vi "Glimpse Plugin Handler.vi"() -> ()   [LabVIEW 2016]
doc: "Select a listed SubVI (stand-alone or inside an .llb) and execute it. Plug-ins run asynchronously from Glimpse (this means that both the plug-in and Glimpse run simultaneously). Be careful about doing 2 things at once if one of the tasks is time-criticial (i.e., image acquisition).\n\nFor a plug-in to be included in the list, it must have the right name and be in the right place:\n-- the name must start with \"GPI-\" and end with \".vi\"\n-- for the executable version of Glimpse, plug-ins must be built into the installer; you can't add them later. (Specifically, the plug-in must be linked into the glimpse build as a dynamic VI to be placed in the installation directory.) The executable version of Glimpse also requres that each plug in be added to the list on the front panel of glimpse plugin list plugins.vi\n-- for the source version, the plug-in is simply placed in the same directory as Glimpse.llb\n\nGlimpse Plugin Handler.vi - created 8-3-05 by Marc Bunin\nmods JG 1/3/06"
panel:
  in  "error in (no error)":errorcluster
  out "stripped path":path
  in  "Execute":bool caption="Runs the selected SubVI and ends execution of the Plugin Handler."
  in  "Available Plug-ins":i32(listbox) caption="Select a VI and press Execute."
  in  "Cancel":bool caption="Stops execution of the Plugin Handler."
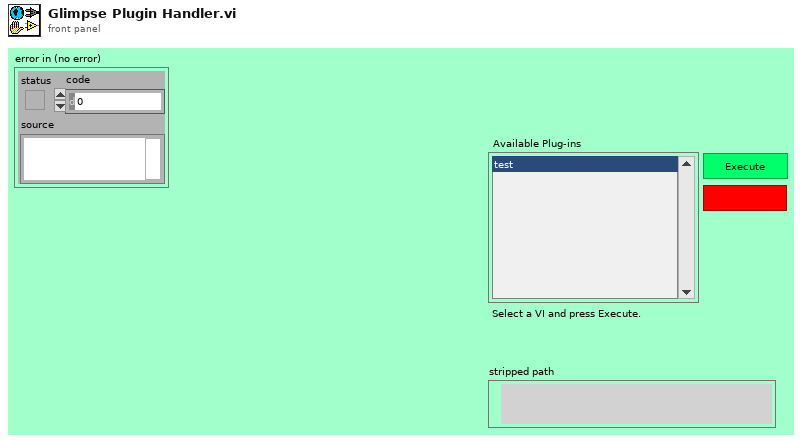
[diagram p1: front panel]
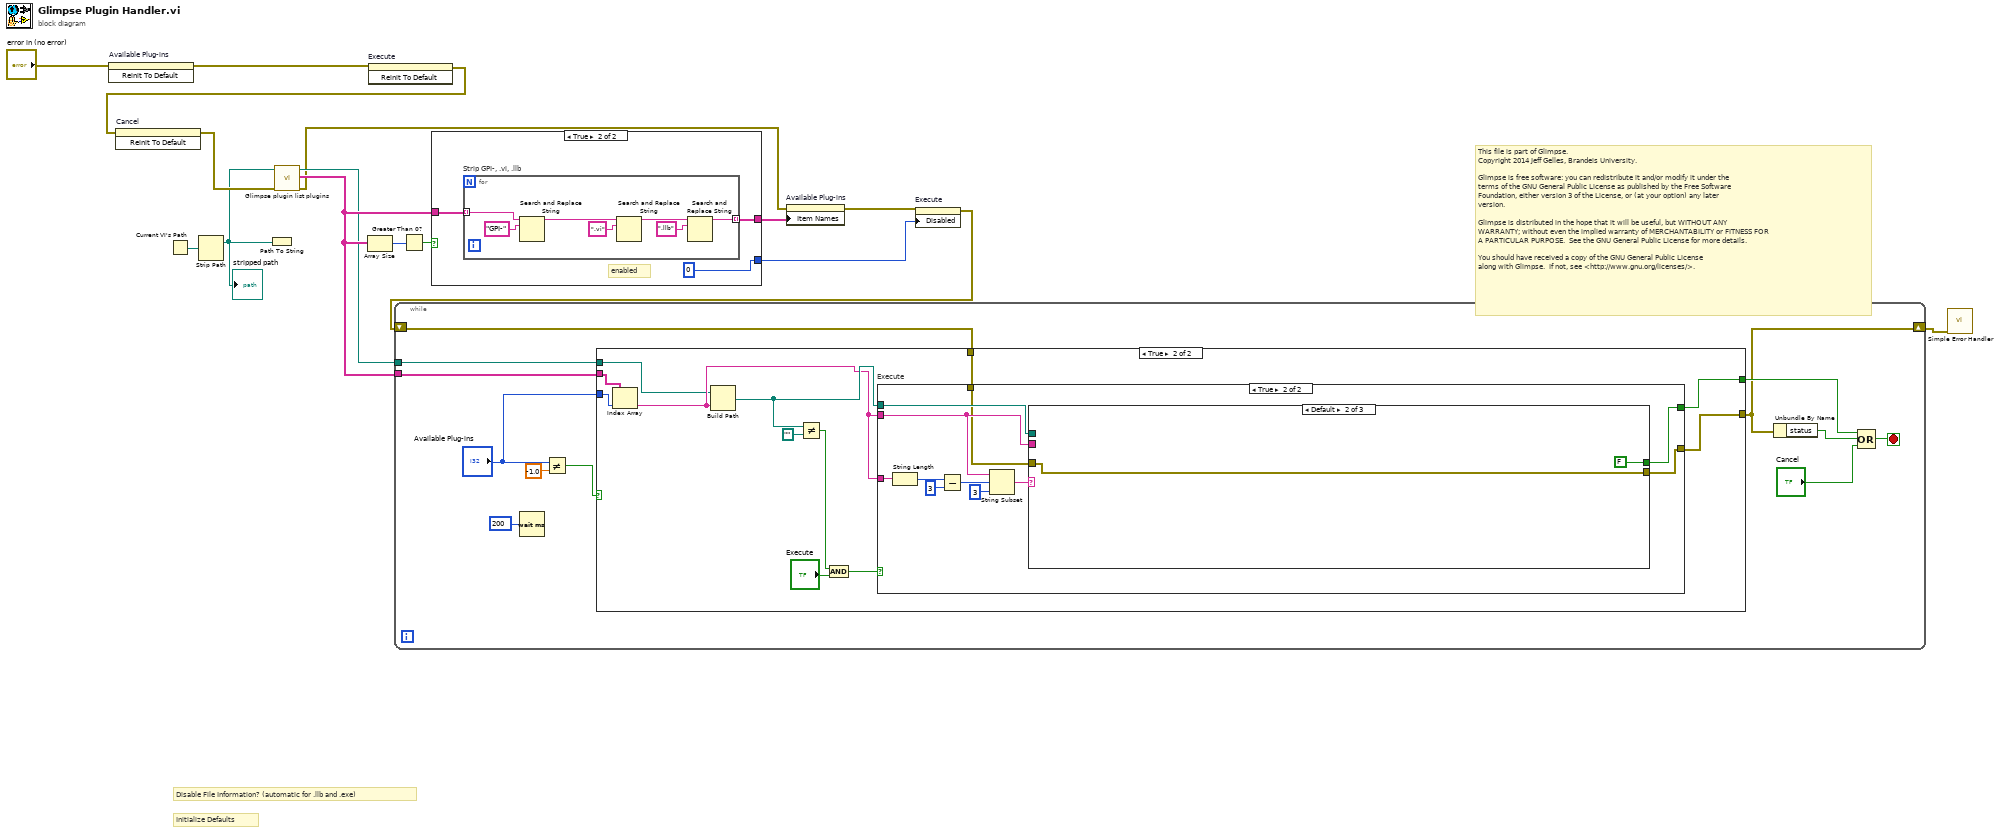
[diagram p0: block diagram]
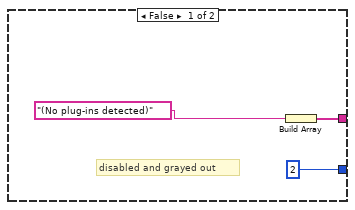
[diagram p2: hidden frame]
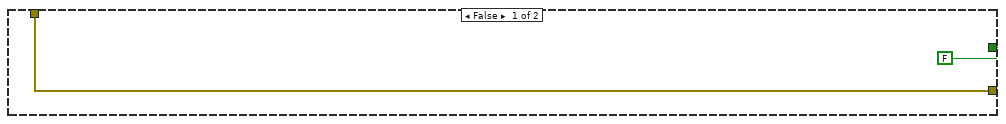
[diagram p3: hidden frame]
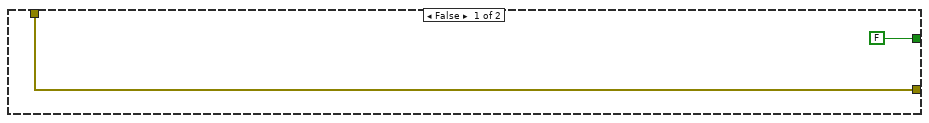
[diagram p4: hidden frame]
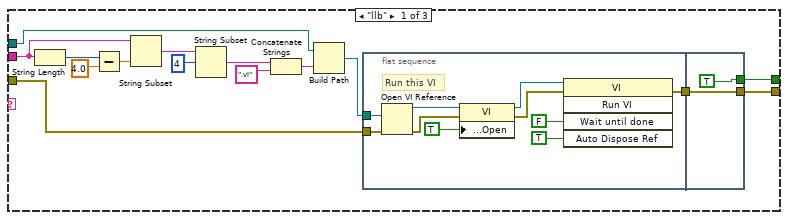
[diagram p5: hidden frame]
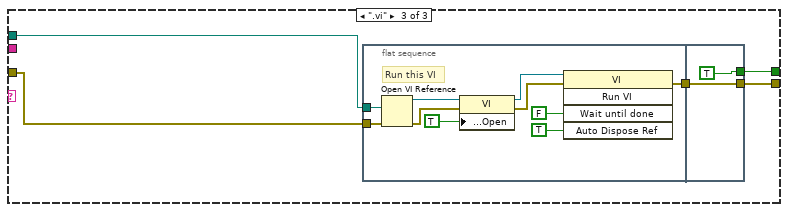
[diagram p6: hidden frame]
diagram:
  # "This file is part of Glimpse. \nCopyright 2014 Jeff Gelles, Brandeis University.    \n\nGlimpse is free software: you can redistribute it and/or modify it under the \nterms of the GNU General Public License as published by the Free Software \nFoundation, either version 3 of the License, or (at your option) any later \nversion.\n\nGlimpse is distributed in the hope that it will be useful, but WITHOUT ANY \nWARRANTY; without even the implied warranty of MERCHANTABILITY or FITNESS FOR \nA PARTICULAR PURPOSE.  See the GNU General Public License for more details.\n\nYou should have received a copy of the GNU General Public License\nalong with Glimpse.  If not, see <http://www.gnu.org/licenses/>."
  # "Disable File Information? (automatic for .llb and .exe)"
  # "Initialize Defaults"
  n1 = invoke on="Available Plug-ins" class="ListBox (strict)" method="Reinit To Default"(error in="error in (no error)") -> (error out=w5:errorcluster)  [unwired: 2 in, 2 out]
  n2 = Current VI's Path() -> (path=w16:path)
  n3 = Strip Path(path=w16) -> (stripped path=w7:path)  [unwired: 1 out]
  "stripped path" <- w7
  n4 = Path To String(path=w7) -> ()  [unwired: 1 out]
  n5 = invoke on="Execute" class="Boolean" method="Reinit To Default"(error in=w5) -> (error out=w15:errorcluster)  [unwired: 2 in, 2 out]
  n6 = invoke on="Cancel" class="Boolean" method="Reinit To Default"(error in=w15) -> (error out=w14:errorcluster)  [unwired: 2 in, 2 out]
  n7 = call "Glimpse plugin list plugins.vi"("error in"=w14, "stripped path"=w7) -> ("error out"=w3:errorcluster, "file names"=w8:string[], "stripped path out"=w6:path)  [unwired: 6 out]
  n8 = Array Size(array=w8) -> (size(s)=w12:i32)
  n9 = Greater Than 0?(x=w12) -> (x > 0?=w11:bool)
  n10 = case shown="True" w11 {
    tunnel: [w19 w22] -> w13
    tunnel: w8 -> [_ w21]
    tunnel: [u8 2 ("Disabled") u8 0 ("Disabled")] -> w10
    frame False {
      # "disabled and grayed out"
      n11 = Build Array("(No plug-ins detected)") -> (w19:string[])
    }
    frame True {
      # "enabled"
      n12 = for "Strip GPI-, .vi, .llb" {
        tunnel: w21 -> [w24] mode=indexing
        tunnel: [w23] -> w22 mode=indexing
        n13 = Search and Replace String(input string=w24, search string="GPI-" ("substring (\"\")")) -> (result string=w28:string)  [unwired: 1 in, 8 out]
        n14 = Search and Replace String(input string=w28, search string=".vi" ("substring (\"\")")) -> (result string=w26:string)  [unwired: 1 in, 8 out]
        n15 = Search and Replace String(input string=w26, search string=".llb") -> (result string=w23:string)  [unwired: 1 in, 8 out]
      }
    }
  }
  n16 = property on="Available Plug-ins" class="LstBox (strict)"(error in=w3, "Item Names"=w13) -> (error out=w9:errorcluster)  [unwired: 1 in, 1 out]
  n17 = property on="Execute" class="Bool"(error in=w9, "Disabled"=w10) -> (error out=w2:errorcluster)  [unwired: 1 in, 1 out]
  n18 = while {
    tunnel: w8 -> [w37]
    tunnel: w6 -> [w36]
    shift-right: [w30] -> w1
    shift-left: w2 -> [w31]
    stop <- w32 stop-if-true
    n19 = Wait (ms)(milliseconds to wait=u32 200) -> ()  [unwired: 1 out]
    n20 = Not Equal?(x="Available Plug-ins", y=-1.0) -> (x != y?=w41:bool)
    n21 = case shown="True" w41 {
      tunnel: "Available Plug-ins" -> [_ w55]
      tunnel: [w42 w49] -> w30
      tunnel: [FALSE w48] -> w33
      tunnel: w37 -> [_ w46]
      tunnel: w36 -> [_ w45]
      tunnel: w31 -> [w42 w44]
      frame False {
      }
      frame True {
        n22 = Index Array ("Selected File (name)")(array=w46, index=w55) -> (element=w47:string)
        n23 = Build Path ("Full File Path")(base path=w45, name or relative path=w47) -> (appended path=w50:path)
        n24 = Not Equal?(x=w50, y=path "") -> (x != y?=w51:bool)
        n25 = And(x=w51, y="Execute") -> (x .and. y?=w53:bool)
        n26 = case "Execute" shown="True" w53 {
          tunnel: w50 -> [_ w68]
          tunnel: [w56 w67] -> w49
          tunnel: [FALSE w66] -> w48
          tunnel: w47 -> [_ w65]
          tunnel: w47 -> [_ w63]
          tunnel: w44 -> [w56 w58]
          frame False {
          }
          frame True {
            n27 = String Length(string=w65) -> (length=w60:i32)
            n28 = Subtract(x=w60, y=3 ("x")) -> (x-y=w61:i32)
            n29 = String Subset(string=w63, offset (0)=w61, length (rest)=3 ("length (rest)")) -> (substring=w64:string)
            n30 = case shown="Default" w64 {
              tunnel: w68 -> [w81 _ w101]
              tunnel: [w73 w96 w100] -> w67
              tunnel: [w82 FALSE w99] -> w66
              tunnel: w63 -> [w80 _ _]
              tunnel: w58 -> [w69 w96 w98]
              frame "llb" {
                n31 = String Length(string=w80) -> (length=w77:i32)
                n32 = Subtract(x=w77, y=4.0) -> (x-y=w78:dbl)
                n33 = String Subset(string=w80, length (rest)=w78) -> (substring=w72:string)  [unwired: 1 out]
                n34 = String Subset(string=w72, offset (0)=4) -> (substring=w70:string)  [unwired: 1 out]
                n35 = Concatenate Strings(w70, ".vi" ("string")) -> (w75:string)
                n36 = Build Path(base path=w81, name or relative path=w75) -> (appended path=w74:path)
                n37 = flat-sequence {
                  tunnel: [w86] -> w83
                  tunnel: w74 -> [w85]
                  tunnel: w69 -> [w84]
                  tunnel: [w95] -> w73
                  tunnel: w83 -> [w95]
                  tunnel: [TRUE] -> w82
                  frame #0 {
                    # "Run this VI"
                    n38 = Open VI Reference(vi path=w85, error in (no error)=w84) -> (vi reference=w93:refnum<vi>, error out=w88:errorcluster)  [unwired: 4 out]
                    n39 = property class="VI"(reference=w93, error in=w88, "Front Panel Window:Open"=TRUE) -> (reference out=w91:refnum<vi>, error out=w87:errorcluster)
                    n40 = invoke class="VI" method="Run VI"(reference=w91, error in=w87, "Wait until done"=FALSE, "Auto Dispose Ref"=TRUE) -> (error out=w86:errorcluster)  [unwired: 1 in, 4 out]
                  }
                  frame #1 {
                  }
                }
              }
              frame Default {
              }
              frame ".vi" {
                n41 = flat-sequence {
                  tunnel: w101 -> [w104]
                  tunnel: [w105] -> w102
                  tunnel: w98 -> [w103]
                  tunnel: [w114] -> w100
                  tunnel: w102 -> [w114]
                  tunnel: [TRUE] -> w99
                  frame #0 {
                    # "Run this VI"
                    n42 = Open VI Reference(vi path=w104, error in (no error)=w103) -> (vi reference=w112:refnum<vi>, error out=w107:errorcluster)  [unwired: 4 out]
                    n43 = property class="VI"(reference=w112, error in=w107, "Front Panel Window:Open"=TRUE) -> (reference out=w110:refnum<vi>, error out=w106:errorcluster)
                    n44 = invoke class="VI" method="Run VI"(reference=w110, error in=w106, "Wait until done"=FALSE, "Auto Dispose Ref"=TRUE) -> (error out=w105:errorcluster)  [unwired: 1 in, 4 out]
                  }
                  frame #1 {
                  }
                }
              }
            }
          }
        }
      }
    }
    n45 = Unbundle By Name(w30) -> ("status"=w35:bool)
    n46 = Compound Arithmetic op=OR(w33, w35, "Cancel") -> (w32:bool)
  }
  n47 = call <vilib>:"Simple Error Handler.vi"("error in (no error)"=w1) -> ()  [unwired: 1 in, 8 out]
